vi "CT_BuildDischargeIdentity.vi"(1 "Cap Discharge Array In":T1=[{"cap number and switch SN array"=[{"Switch SN"="SN_U", "Cap Number"=109.0}], "Rog"=enum."F240", "Delay"=enum."PreForm", "Power Supply"=enum."PS1"}, {"cap number and switch SN array"=[{"Switch SN"="SN_U", "Cap Number"=110.0}], "Rog"=enum."F180", "Delay"=enum."DB16", "Power Supply"=enum."PS2"}, {"cap number and switch SN array"=[{"Switch SN"="SN_U", "Cap Number"=111.0}], "Rog"=enum."F300", "Delay"=enum."DB16", "Power Supply"=enum."PS2"}, {"cap number and switch SN array"=[{"Switch SN"="SN_U", "Cap Number"=112.0}], "Rog"=enum."F000", "Delay"=enum."DB16", "Power Supply"=enum."PS2"}, {"cap number and switch SN array"=[{"Switch SN"="SN_U", "Cap Number"=113.0}], "Rog"=enum."F060", "Delay"=enum."DB16", "Power Supply"=enum."PS2"}, {"cap number and switch SN array"=[{"Switch SN"="SN_U", "Cap Number"=114.0}], "Rog"=enum."F120", "Delay"=enum."DB16", "Power Supply"=enum."PS2"}, {"cap number and switch SN array"=[{"Switch SN"="SN_U", "Cap Number"=115.0}], "Rog"=enum."F120", "Delay"=enum."DB16", "Power Supply"=enum."PS2"}, {"cap number and switch SN array"=[{"Switch SN"="SN_U", "Cap Number"=116.0}], "Rog"=enum."F060", "Delay"=enum."DB16", "Power Supply"=enum."PS2"}, {"cap number and switch SN array"=[{"Switch SN"="SN_U", "Cap Number"=117.0}], "Rog"=enum."F000", "Delay"=enum."DB16", "Power Supply"=enum."PS2"}, {"cap number and switch SN array"=[{"Switch SN"="SN_U", "Cap Number"=118.0}], "Rog"=enum."F300", "Delay"=enum."DB16", "Power Supply"=enum."PS2"}, {"cap number and switch SN array"=[{"Switch SN"="SN_U", "Cap Number"=119.0}], "Rog"=enum."F180", "Delay"=enum."DB16", "Power Supply"=enum."PS2"}, {"cap number and switch SN array"=[{"Switch SN"="SN_U", "Cap Number"=120.0}], "Rog"=enum."F240", "Delay"=enum."DB16", "Power Supply"=enum."PS2"}, {"cap number and switch SN array"=[{"Switch SN"="SN_U", "Cap Number"=121.0}], "Rog"=enum."F240", "Delay"=enum."DB16", "Power Supply"=enum."PS3"}, {"cap number and switch SN array"=[{"Switch SN"="SN_U", "Cap Number"=122.0}], "Rog"=enum."F300", "Delay"=enum."DB16", "Power Supply"=enum."PS3"}, {"cap number and switch SN array"=[{"Switch SN"="SN_U", "Cap Number"=123.0}], "Rog"=enum."F180", "Delay"=enum."DB16", "Power Supply"=enum."PS3"}, {"cap number and switch SN array"=[{"Switch SN"="SN_U", "Cap Number"=124.0}], "Rog"=enum."F240", "Delay"=enum."DB16", "Power Supply"=enum."PS3"}, {"cap number and switch SN array"=[{"Switch SN"="SN_U", "Cap Number"=125.0}], "Rog"=enum."DISC", "Delay"=enum."DB16", "Power Supply"=enum."PS3"}, {"cap number and switch SN array"=[{"Switch SN"="SN_U", "Cap Number"=126.0}], "Rog"=enum."F000", "Delay"=enum."DB16", "Power Supply"=enum."PS3"}, {"cap number and switch SN array"=[{"Switch SN"="SN_U", "Cap Number"=127.0}], "Rog"=enum."F060", "Delay"=enum."DB16", "Power Supply"=enum."PS3"}, {"cap number and switch SN array"=[{"Switch SN"="SN_U", "Cap Number"=128.0}], "Rog"=enum."DISC", "Delay"=enum."DB16", "Power Supply"=enum."PS3"}]) -> (0 "Discharge Identity":string[][](array[string]))   [LabVIEW 2016]
uses:
  CapDischargeCluster.ctl
panel:
  out "size(s)":i32[](array[numeric])
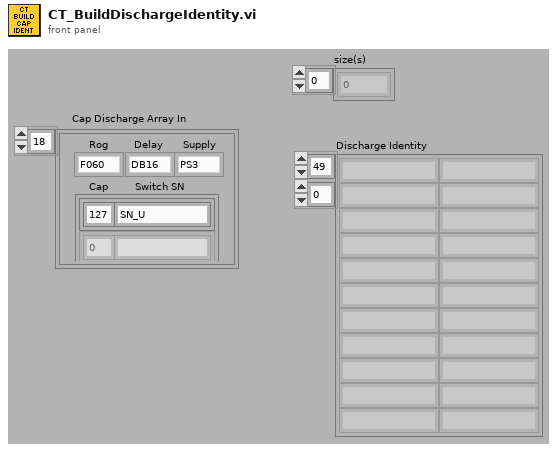
[diagram p1: front panel]
types:
  T1 = typedef "CapDischargeCluster.ctl" = cluster{"cap number and switch SN array":cluster{"Switch SN":string, "Cap Number":dbl}[], "Rog":enum16{"F000", "F060", "F120", "F180", "F240", "F300", "A015", "A045", "A075", "A105", "A135", "A165", "A195", "A225", "A255", "A285", "A315", "A345", "Snip", "DISC"}, "Delay":enum16{"DB00", "DB01", "DB02", "DB03", "DB04", "DB05", "DB06", "DB07", "DB08", "DB09", "DB10", "DB11", "DB12", "DB13", "DB14", "DB15", "DB16", "DB17", "DB18", "DB19", "DB20", "DB21", "DB22", "DB23", "DB24", "DB25", "DB26", "DB27", "DB28", "DB29", "DB30", "PreForm", "Form"}, "Power Supply":enum16{"PS1", "PS2", "PS3", "PS5", "PS6", "PS4"}}[]
  T2 = enum16{"F000", "F060", "F120", "F180", "F240", "F300", "A015", "A045", "A075", "A105", "A135", "A165", "A195", "A225", "A255", "A285", "A315", "A345", "Snip", "DISC"}
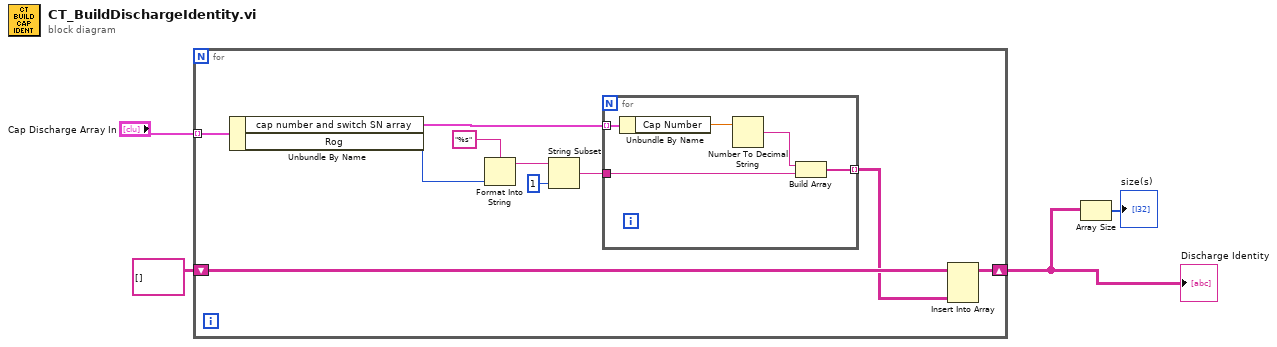
[diagram p0: block diagram]
diagram:
  n1 = for {
    tunnel: "Cap Discharge Array In" -> [w14] mode=indexing
    shift-right: [w5] -> w3
    shift-left: string[][] [] -> [w7]
    n2 = Unbundle By Name(w14) -> ("cap number and switch SN array"=w13:cluster{"Switch SN":string, "Cap Number":dbl}[], "Rog"=w12:T2)
    n3 = Format Into String(format string="%s", w12) -> (resulting string=w10:string)  [unwired: 2 in, 1 out]
    n4 = String Subset(string=w10, length (rest)=1 ("length (rest)")) -> (substring=w8:string)  [unwired: 1 in]
    n5 = for {
      tunnel: w13 -> [w19] mode=indexing
      tunnel: w8 -> [w17]
      tunnel: [w15] -> w6 mode=indexing
      n6 = Unbundle By Name(w19) -> ("Cap Number"=w18:dbl)
      n7 = Number To Decimal String(number=w18) -> (decimal integer string=w16:string)  [unwired: 1 in]
      n8 = Build Array(w16, w17) -> (w15:string[])
    }
    n9 = Insert Into Array(array=w7, new element=w6) -> (w5:string[][])  [unwired: 2 in]
  }
  "Discharge Identity" <- w3
  n10 = Array Size(array=w3) -> (size(s)=→"size(s)":i32[])
